vi "Read Top Right.vi"(8 "error in (no error)":errorcluster, 11 "Tool Rectangle in":refnum<class "Tool Rectangle.lvclass">) -> (0 "error out":errorcluster, 2 "Top Right":cluster{"X":dbl, "Y":dbl}, 3 "Tool Rectangle out":refnum<class "Tool Rectangle.lvclass">)   [LabVIEW 2019, in "Tool Rectangle.lvclass"]
uses:
  Tool Rectangle.lvclass
  Tool Rectangle.lvclass/Tool Rectangle.ctl
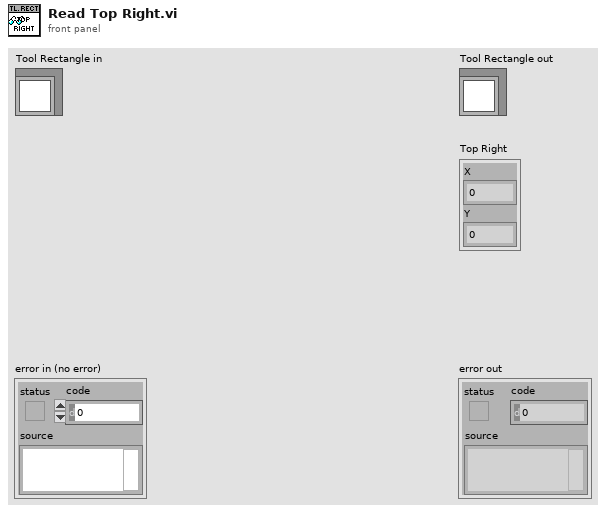
[diagram p1: front panel]
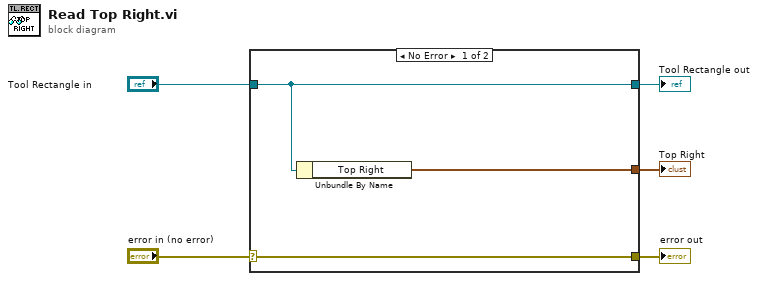
[diagram p0: block diagram]
diagram:
  n1 = case shown="No Error" "error in (no error)" {
    selector: "error in (no error)" -> [w8 w9]
    tunnel: [w8 w9] -> w4
    tunnel: [w7 w10] -> w2
    tunnel: "Tool Rectangle in" -> [w7 w10]
    tunnel: [w6 _] -> w1
    frame No Error {
      n2 = Unbundle By Name(w7) -> ("Top Right"=w6:cluster{"X":dbl, "Y":dbl})
    }
    frame Error {
    }
  }
  "error out" <- w4
  "Tool Rectangle out" <- w2
  "Top Right" <- w1
